vi "Case Structures.vi"() -> ()   [LabVIEW 2012]
panel:
  out "Random Value":dbl
  in  "error in (no error)":errorcluster
  in  "Enum Selection":enum16{"Option A", "Option B", "Option C"}(ring)
  in  "String Selection":string
  in  "Numeric Selection":i32
  in  "Boolean Selection":bool
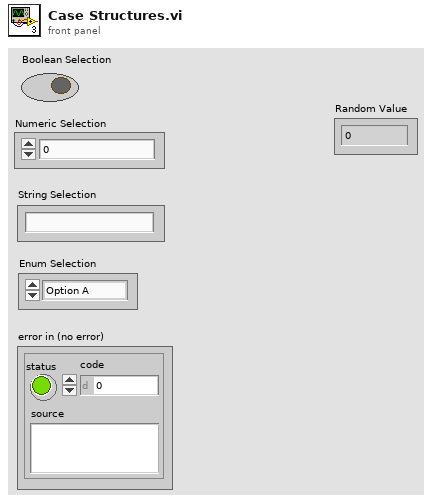
[diagram p1: front panel]
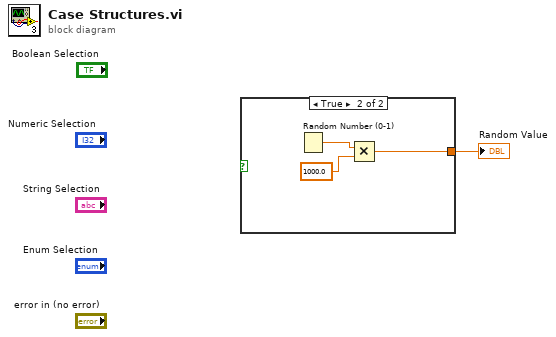
[diagram p0: block diagram]
diagram:
  n1 = case shown="True" {
    selector: _ -> [_ _]
    tunnel: [_ w2] -> w1
    frame False {
    }
    frame True {
      n2 = Random Number (0-1)() -> (number: 0 to 1=w4:dbl)
      n3 = Multiply(x=w4, y=1000.0) -> (x*y=w2:dbl)
    }
  }
  "Random Value" <- w1
